vi "teste retro action.vi"() -> ()   [LabVIEW 2026]
uses:
  C:/Users/laserfab/Desktop/T-Cube TPZ001-LV2026Q1/Thorlabs.MotionControl.Controls.dll
  Thorlabs.MotionControl.Controls.dll
  C:/Users/laserfab/Desktop/T-Cube TPZ001-LV2026Q1/Thorlabs.MotionControl.TCube.PiezoCLI.dll
  Thorlabs.MotionControl.TCube.PiezoCLI.dll
  <vilib>/numeric/Random Number (Range) DBL.vi
panel:
  in  "stop 2":bool
  out "CentroidY":dbl format="%#_6f"
  out "error out":errorcluster caption="sortie d'erreur"
  in  "error in (no error)":errorcluster caption="entrée d'erreur (pas d'erreur)"
  in  "ROI":dbl[][](array[numeric])
  out "CentroidX":dbl format="%#_6f"
  out "CloseDevice 2":bool=TRUE
  in  "SerialNumber 2":string="81844656"
  out "GetOutputVoltage 2":dbl=0.00686666463209937
  out "CreateDevice 2":bool=TRUE
  in  "TCubePiezoControl 2":refnum<k24>(container)
  out "CloseDevice":bool=TRUE
  in  "stop":bool
  out "GetOutputVoltage":dbl=0.00686666463209937
  out "CreateDevice":bool=TRUE
  in  "SerialNumber":string="81844665"
  in  "TCubePiezoControl":refnum<k24>(container)
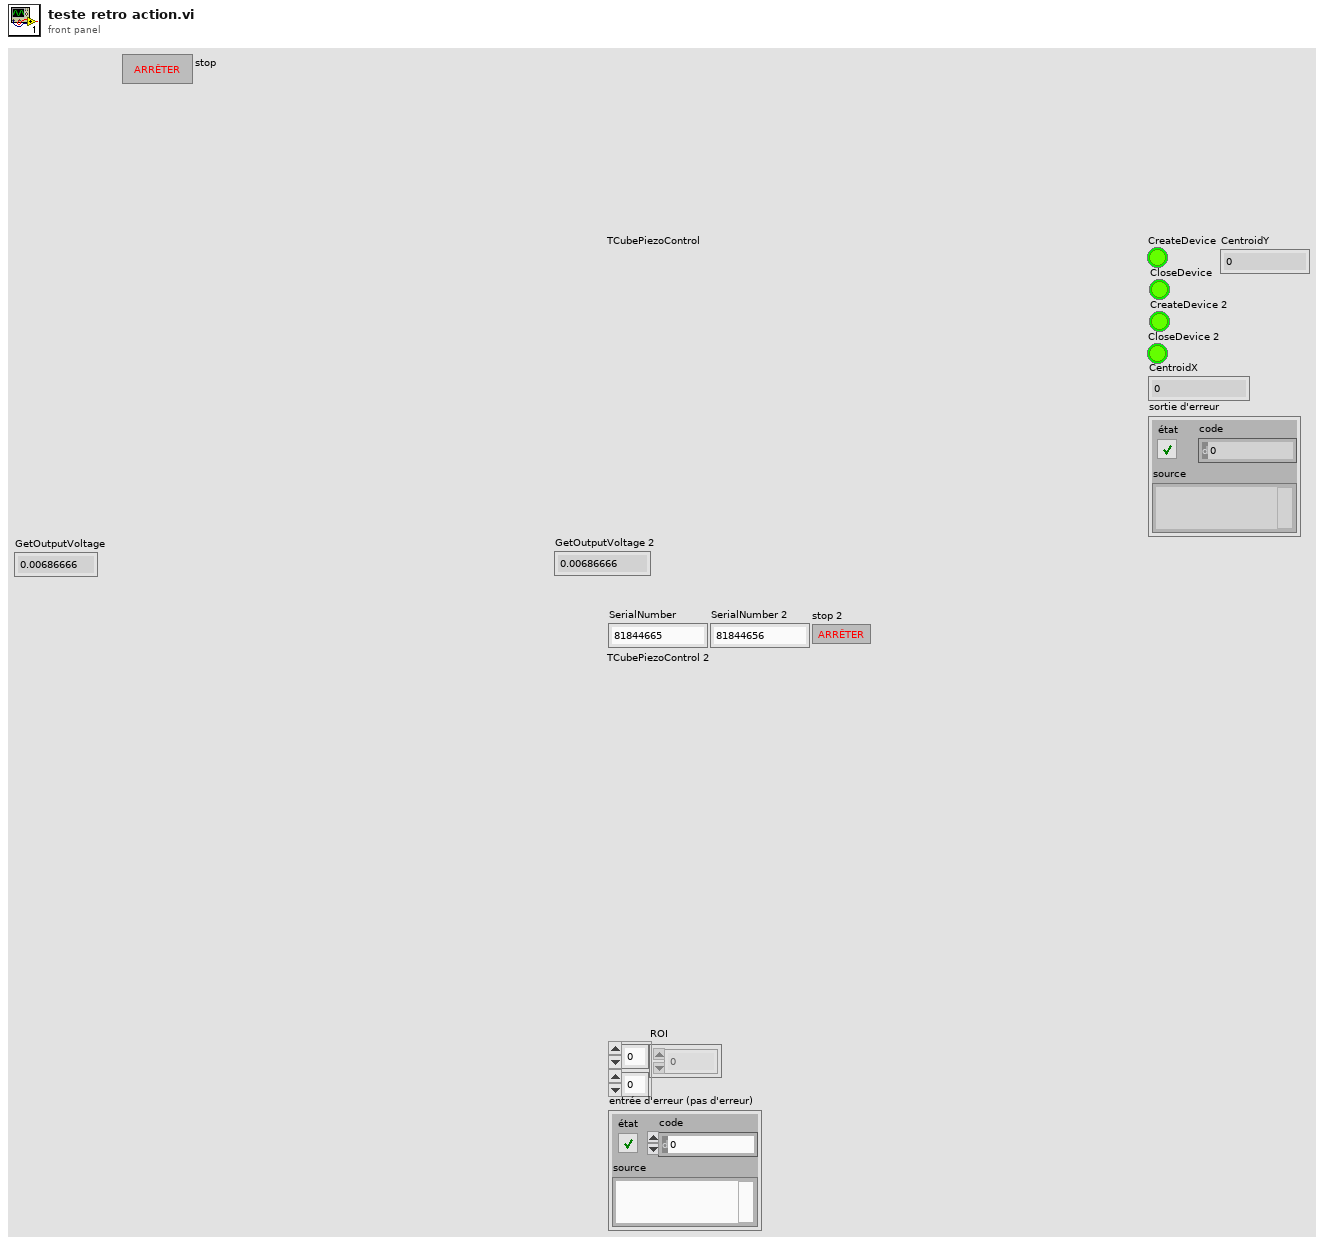
[diagram p1: front panel]
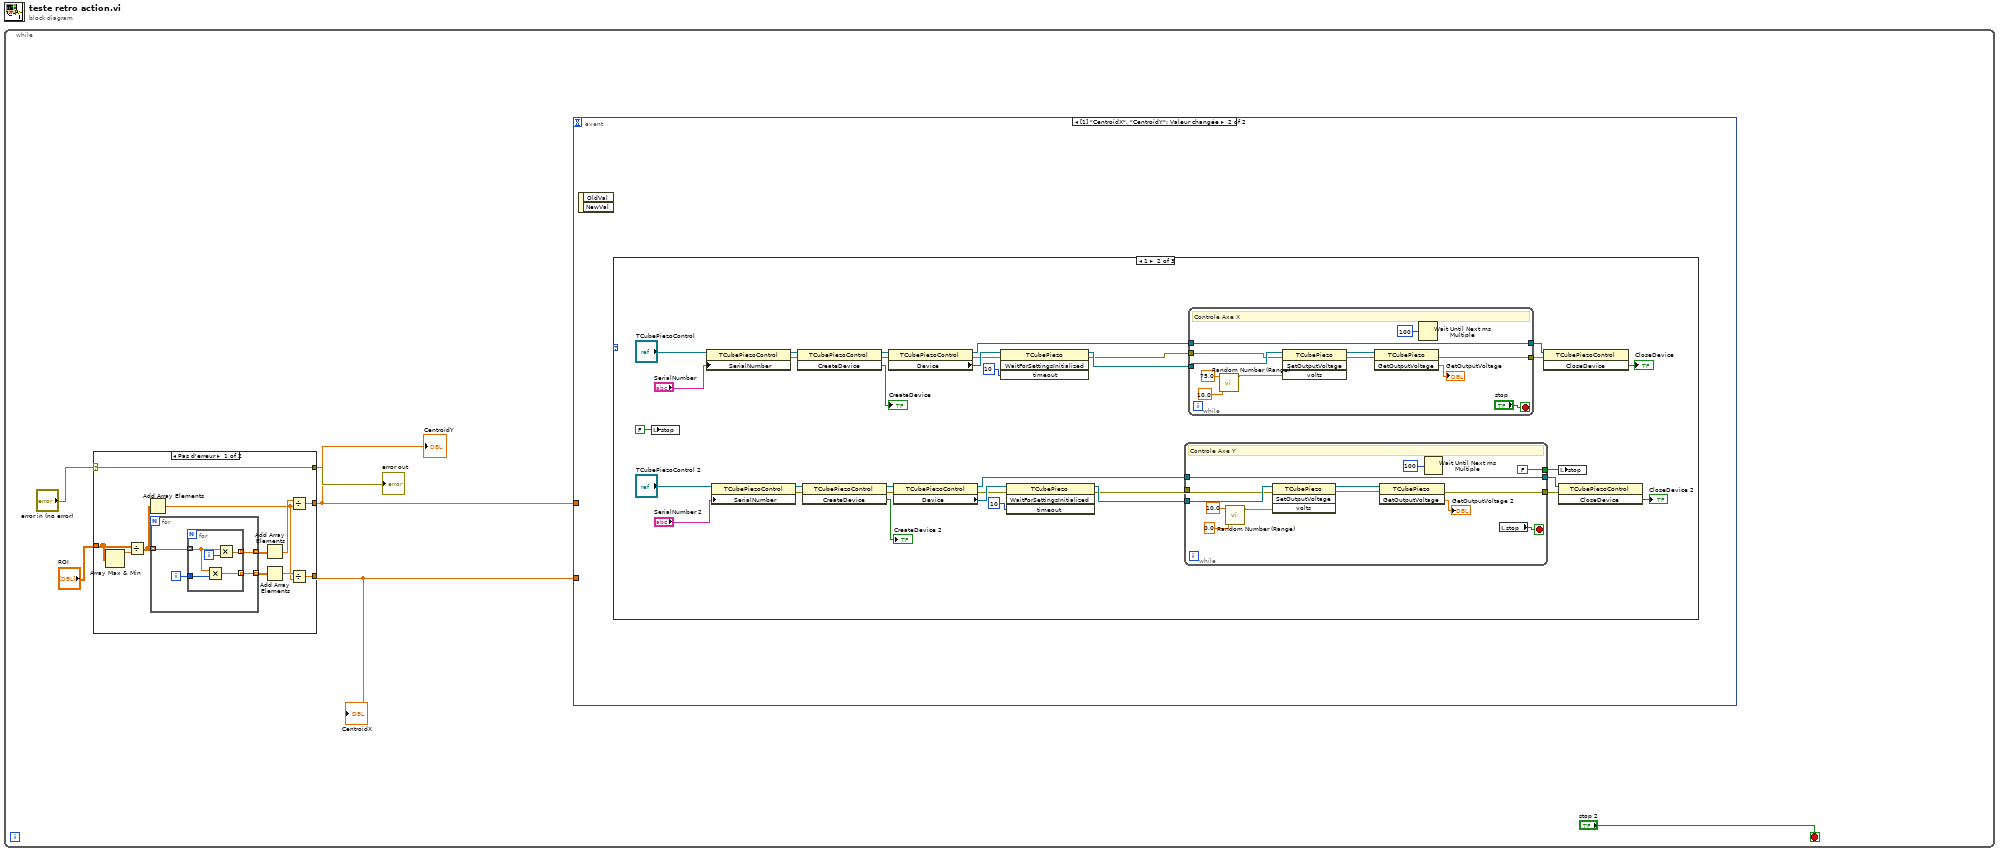
[diagram p0: block diagram]
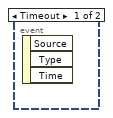
[diagram p3: hidden frame]
diagram:
  n1 = while {
    stop <- "stop 2" stop-if-true
    n2 = case shown="Pas d'erreur" "error in (no error)" {
      selector: "error in (no error)" -> [w7 w27]
      tunnel: [w14 _] -> w2
      tunnel: "ROI" -> [w10 _]
      tunnel: [w8 _] -> w1
      tunnel: [w7 w27] -> w5
      frame No Error {
        n3 = Array Max & Min(array=w10) -> (max value=w11:dbl)  [unwired: 3 out]
        n4 = Divide(x=w10, y=w11) -> (x/y=w9:dbl[][])
        n5 = Add Array Elements(numeric array=w9) -> (sum=w12:dbl)
        n6 = for {
          tunnel: w9 -> [w20] mode=indexing
          tunnel: [w19] -> w17 mode=indexing
          tunnel: [w18] -> w15 mode=indexing
          i -> [w21]
          n7 = for {
            tunnel: w21 -> [w26]
            tunnel: w20 -> [w22] mode=indexing
            tunnel: [w25] -> w19 mode=indexing
            tunnel: [w23] -> w18 mode=indexing
            i -> [w24]
            n8 = Multiply(x=w22, y=w26) -> (x*y=w25:dbl)
            n9 = Multiply(x=w22, y=w24) -> (x*y=w23:dbl)
          }
        }
        n10 = Add Array Elements(numeric array=w15) -> (sum=w13:dbl)
        n11 = Add Array Elements(numeric array=w17) -> (sum=w16:dbl)
        n12 = Divide(x=w13, y=w12) -> (x/y=w8:dbl)
        n13 = Divide(x=w16, y=w12) -> (x/y=w14:dbl)
      }
      frame Error {
      }
    }
    "CentroidX" <- w2
    "error out" <- w5
    "CentroidY" <- w1
    n14 = event shown="[1] \"CentroidX\", \"CentroidY\": Valeur changée" {
      selector: _ -> [_ _]
      dyn-events: _ -> [_ _]
      timeout: _ -> [_ _]
      tunnel: w2 -> [_ _]
      tunnel: w1 -> [_ _]
      event Timeout {
        n15 = event-data() -> ()  [unwired: 1 in, 3 out]
      }
      event "CentroidX", "CentroidY": Value Change {
        n16 = event-data() -> ()  [unwired: 1 in, 2 out]
        n17 = case shown="1" {
          selector: _ -> [_ _ _]
          frame 0, Default {
          }
          frame 1 {
            n18 = local write "stop"(FALSE ("stop")) -> ()
            n19 = property on="Nœud de propriété" class="TCubePiezoControl"(reference="TCubePiezoControl", "SerialNumber"="SerialNumber") -> (reference out=w59:refnum<k24>, error out=w58:errorcluster)  [unwired: 1 in]
            n20 = property on="Nœud de propriété" class="TCubePiezoControl"(reference="TCubePiezoControl 2", "SerialNumber"="SerialNumber 2") -> (reference out=w50:refnum<k24>, error out=w49:errorcluster)  [unwired: 1 in]
            n21 = invoke on="Nœud de méthode" class="TCubePiezoControl" method="CreateDevice"(reference=w59, error in=w58) -> (reference out=w56:refnum<k24>, error out=w57:errorcluster, "CreateDevice"=→"CreateDevice":bool)  [unwired: 1 in]
            n22 = invoke on="Nœud de méthode" class="TCubePiezoControl" method="CreateDevice"(reference=w50, error in=w49) -> (reference out=w47:refnum<k24>, error out=w48:errorcluster, "CreateDevice"=→"CreateDevice 2":bool)  [unwired: 1 in]
            n23 = property on="Nœud de propriété" class="TCubePiezoControl"(reference=w56, error in=w57) -> (reference out=w54:refnum<k24>, error out=w35:errorcluster, "Device"=w36:refnum<k24>)
            n24 = property on="Nœud de propriété" class="TCubePiezoControl"(reference=w47, error in=w48) -> (reference out=w45:refnum<k24>, error out=w37:errorcluster, "Device"=w38:refnum<k24>)
            n25 = invoke on="Nœud de méthode" class="TCubePiezo" method="WaitForSettingsInitialized"(reference=w36, error in=w35, "timeout"=10) -> (reference out=w34:refnum<k24>, error out=w33:errorcluster)  [unwired: 1 in, 2 out]
            n26 = invoke on="Nœud de méthode" class="TCubePiezo" method="WaitForSettingsInitialized"(reference=w38, error in=w37, "timeout"=10) -> (reference out=w32:refnum<k24>, error out=w31:errorcluster)  [unwired: 1 in, 2 out]
            n27 = while {
              tunnel: w45 -> [w74]
              tunnel: [w74] -> w44
              tunnel: [w73] -> w43
              tunnel: [FALSE ("stop")] -> w39
              tunnel: w32 -> [w68]
              tunnel: w31 -> [w67]
              stop <- w70 stop-if-true
              # "Controle Axe Y"
              n28 = call-poly <vilib>:"Random Number (Range).vi"("lower bound (0)"=0.0, "upper bound (100)"=10.0) -> ("number"=w63:dbl)  [unwired: 9 in]
              n29 = invoke on="Nœud de méthode" class="TCubePiezo" method="SetOutputVoltage"(reference=w68, error in=w67, "volts"=w63) -> (reference out=w66:refnum<k24>, error out=w65:errorcluster)  [unwired: 1 in, 2 out]
              n30 = invoke on="Nœud de méthode" class="TCubePiezo" method="GetOutputVoltage"(reference=w66, error in=w65) -> (error out=w73:errorcluster, "GetOutputVoltage"=→"GetOutputVoltage 2":dbl)  [unwired: 1 in, 1 out]
              n31 = Wait Until Next ms Multiple(millisecond multiple=u32 100 ("n millisecondes")) -> ()  [unwired: 1 out]
              n32 = local read "stop"() -> (w70:bool)
            }
            n33 = while {
              tunnel: w54 -> [w86]
              tunnel: [w86] -> w53
              tunnel: [w85] -> w52
              tunnel: w34 -> [w81]
              tunnel: w33 -> [w80]
              stop <- "stop" stop-if-true
              # "Controle Axe X"
              n34 = call-poly <vilib>:"Random Number (Range).vi"("lower bound (0)"=10.0, "upper bound (100)"=75.0) -> ("number"=w76:dbl)  [unwired: 9 in]
              n35 = invoke on="Nœud de méthode" class="TCubePiezo" method="SetOutputVoltage"(reference=w81, error in=w80, "volts"=w76) -> (reference out=w79:refnum<k24>, error out=w78:errorcluster)  [unwired: 1 in, 2 out]
              n36 = invoke on="Nœud de méthode" class="TCubePiezo" method="GetOutputVoltage"(reference=w79, error in=w78) -> (error out=w85:errorcluster, "GetOutputVoltage"=→"GetOutputVoltage":dbl)  [unwired: 1 in, 1 out]
              n37 = Wait Until Next ms Multiple(millisecond multiple=u32 100 ("n millisecondes")) -> ()  [unwired: 1 out]
            }
            n38 = invoke on="Nœud de méthode" class="TCubePiezoControl" method="CloseDevice"(reference=w53, error in=w52) -> ("CloseDevice"=→"CloseDevice":bool)  [unwired: 1 in, 2 out]
            n39 = local write "stop"(w39) -> ()
            n40 = invoke on="Nœud de méthode" class="TCubePiezoControl" method="CloseDevice"(reference=w44, error in=w43) -> ("CloseDevice"=→"CloseDevice 2":bool)  [unwired: 1 in, 2 out]
          }
          frame 2 {
          }
        }
      }
    }
  }
